vi "LMS Sim Vector 5.vi"(8 "Sim Course":i8[][](array[numeric]), 9 "Robot Heading":dbl, 10 "Robot Long":dbl=81.2675 format="%#_8g", 11 "Robot Lat":dbl=37.1526 format="%#_8g") -> (3 "dist":i32[](array[numeric]))   [LabVIEW 2014]
panel:
  # "Inputs:"
  # "Output:"
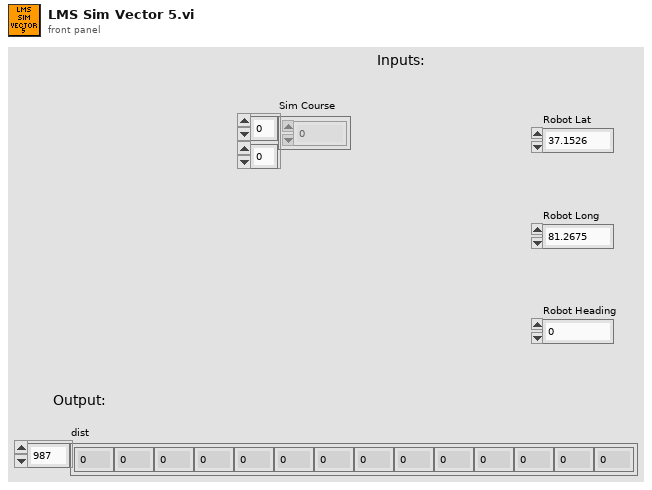
[diagram p1: front panel]
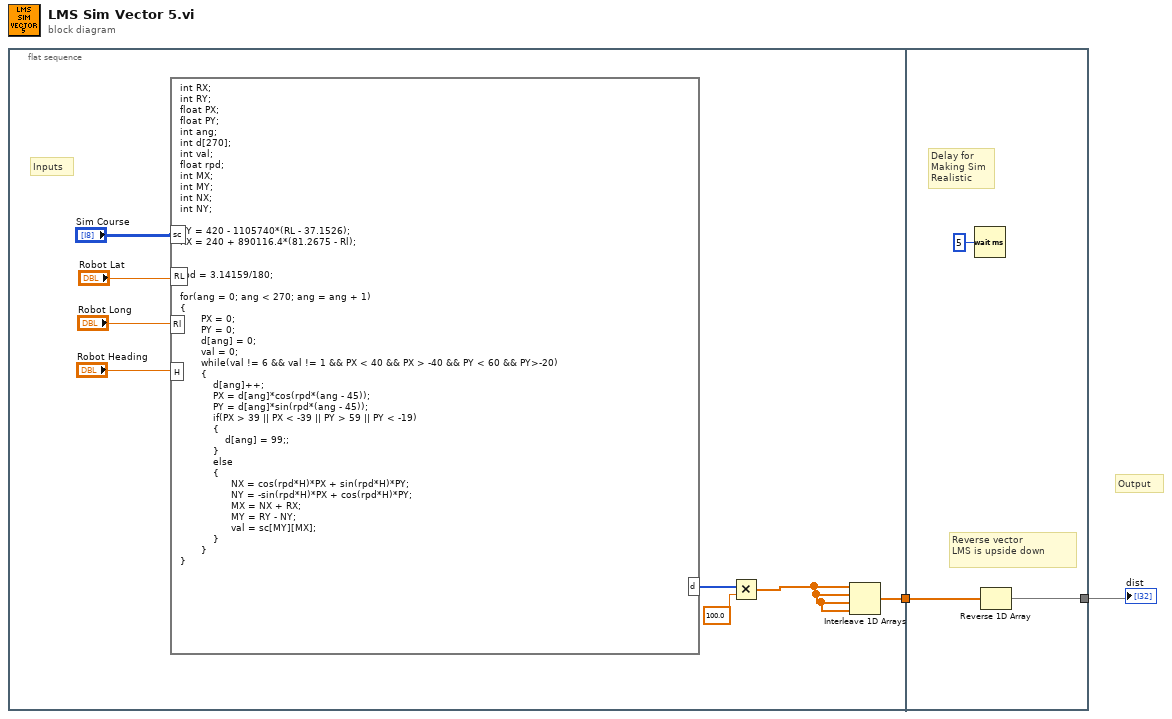
[diagram p0: block diagram]
diagram:
  # "Output"
  n1 = flat-sequence {
    tunnel: [w7] -> w1
    tunnel: [w11] -> w2
    tunnel: w1 -> [w12]
    frame #0 {
      # "Inputs"
      n2 = formula code="int RX;\nint RY;\nfloat PX;\nfloat PY;\nint ang;\nint d[270];\nint val;\nfloat rpd;\nint MX;\nint MY;\nint NX;\nint NY;\n\nRY = 420 - 1105740*(RL - 37.1526);\nRX = 240 + 890116.4*(81.2675 - Rl);\n\n\nrpd = 3.14159/180;\n\nfor(ang = 0; ang < 270; ang = ang + 1)\n{\n       PX = 0;\n       PY = 0;\n       d[ang] = 0;\n       val = 0;\n       while(val != 6 && val != 1 && PX < 40 && PX > -40 && PY < 60 && PY>-20) \n       {\n           d[ang]++;\n           PX = d[ang]*cos(rpd*(ang - 45));\n           PY = d[ang]*sin(rpd*(ang - 45));\n           if(PX > 39 || PX < -39 || PY > 59 || PY < -19)\n           {\n               d[ang] = 99;;\n           }\n           else\n           {\n                 NX = cos(rpd*H)*PX + sin(rpd*H)*PY;\n                 NY = -sin(rpd*H)*PX + cos(rpd*H)*PY;\n                 MX = NX + RX;\n                 MY = RY - NY;\n                 val = sc[MY][MX];\n           }\n       }\n}"("sc"="Sim Course", "RL"="Robot Lat", "Rl"="Robot Long", "H"="Robot Heading") -> ("d"=w4:i32[])
      n3 = Multiply(x=w4, y=100.0) -> (x*y=w6:dbl[])
      n4 = Interleave 1D Arrays(w6, w6, w6, w6) -> (w7:dbl[])
    }
    frame #1 {
      # "Reverse vector\nLMS is upside down"
      # "Delay for\nMaking Sim\nRealistic"
      n5 = Wait (ms)(milliseconds to wait=u32 5) -> ()  [unwired: 1 out]
      n6 = Reverse 1D Array(array=w12) -> (reversed array=w11:dbl[])
    }
  }
  "dist" <- w2
